vi "To Unix Milliseconds.vi"(10 "Time Stamp (Now)":timestamp format="%<%x %.3X>T") -> (2 "Unix Milliseconds":dbl)   [LabVIEW 2020, in "client.lvlib"]
uses:
  client.lvlib
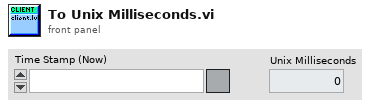
[diagram p1: front panel]
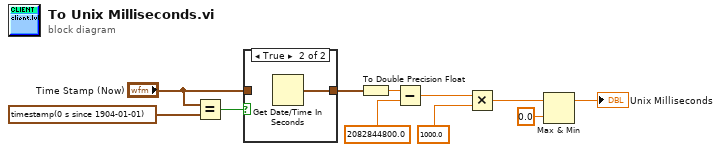
[diagram p0: block diagram]
diagram:
  n1 = Equal?(x="Time Stamp (Now)", y=timestamp(0 s since 1904-01-01) ("Time Stamp")) -> (x = y?=w3:bool)
  n2 = case shown="True" w3 {
    tunnel: "Time Stamp (Now)" -> [w12 _]
    tunnel: [w12 w13] -> w1
    frame False {
    }
    frame True {
      n3 = Get Date/Time In Seconds() -> (seconds since 1Jan1904=w13:timestamp)
    }
  }
  n4 = To Double Precision Float(number=w1) -> (double precision float=w11:dbl)
  n5 = Subtract(x=w11, y=2082844800.0) -> (x-y=w9:dbl)
  n6 = Multiply(x=w9, y=1000.0) -> (x*y=w6:dbl)
  n7 = Max & Min(x=w6, y=0.0) -> (max(x,y)=→"Unix Milliseconds":dbl)  [unwired: 1 out]
